vi "Test Bench v19 - TDMS.vi"() -> ()   [LabVIEW 2022 SP3]
doc: "Use this template to build a producer/consumer design pattern. Use this template when you need to execute a process, such as data analysis, when a data source, such as a triggered acquisition, produces data at an uneven rate and you need to execute the process when the data becomes available."
uses:
  <vilib>/Utility/error.llb/DialogType.ctl
  <vilib>/platform/TimedLoop/XDataNode/XDataNode.xnode
  <vilib>/Platform/TimedLoop/XDataNode/nitl_modes.ctl
  <vilib>/Platform/TimedLoop/XDataNode/XDNodeRunTimeDep.lvlib
  <vilib>/Platform/TimedLoop/XDataNode/wakeup.ctl
  <vilib>/Platform/TimedLoop/XDataNode/timing_clust.ctl
  <vilib>/measure/NI_MAPro.lvlib
  <vilib>/measure/maspectr.llb/FFT Spectrum (Mag-Phase) for 1 Chan.vi
  WhiteNoise.ctl
panel:
  in  "samples per channel":i32=41200
  in  "Folder to save file to":path=path "C:/Users/LAV-UFSC-2023/Documents/LAV-TCC/Dados-Experimentos/Dados-Bancada-LABVIEW"
  out "# pending insert":i32
  out "# pending remove":i32
  out "# elements in queue":i32
  out "Processor 2":i32=-2
  out "Iteration Duration":i64
  out "Processor":i32=-2
  out "Accelerometer":waveform(dbl)(graph)
  out "New file path":path
  in  "Log Data":bool=TRUE
  in  "view":T1={"dB On (F)"=FALSE, "unwrap phase (F)"=TRUE, "convert to degree (F)"=TRUE}
  out "FFT - Phase":cluster{"f0":dbl, "df":dbl, "phase":dbl[]}(graph)
  out "FFT - Magnitude":cluster{"f0":dbl, "df":dbl, "magnitude":dbl[]}(graph)
  out "Signal Output (V)":waveform(dbl)(graph)
  out "Iteration Duration 2":i64
  in  "Enable Output":bool=TRUE
  in  "Signal Output\nControl":enum32{"White Noise", "Harmonic"}(tab)
  in  "White Noise\nParameters":T3={"Seed"=0.0, "Standard Deviation"=2.0, "Reset"=FALSE, "Iterator"=1.0, "Lower Cut-Off"=5.0, "Upper Cut-Off"=350.0} {"Upper Cut-Off" min=5.0 max=350.0 step=10.0; "Lower Cut-Off" min=5.0 max=350.0 step=10.0; "Standard Deviation" min=0.001 max=3.0 step=0.05 format="%0.2p"}
  in  "Hamonic\nParameters":T4={"Waveform Type"=0, "Frequency (Hz)"=10.0, "Amplitude"=0.25} {"Frequency (Hz)" min=5.0 max=350.0 step=10.0 format="%0.2p"; "Waveform Type" items=["Sine Wave", "Triangle Wave", "Square Wave", "Sawtooth Wave"]; "Amplitude" min=0.001 max=0.3 step=0.05 format="%0.2p"}
  in  "stop":bool
  # "Debug Pannel"
  # "Filter"
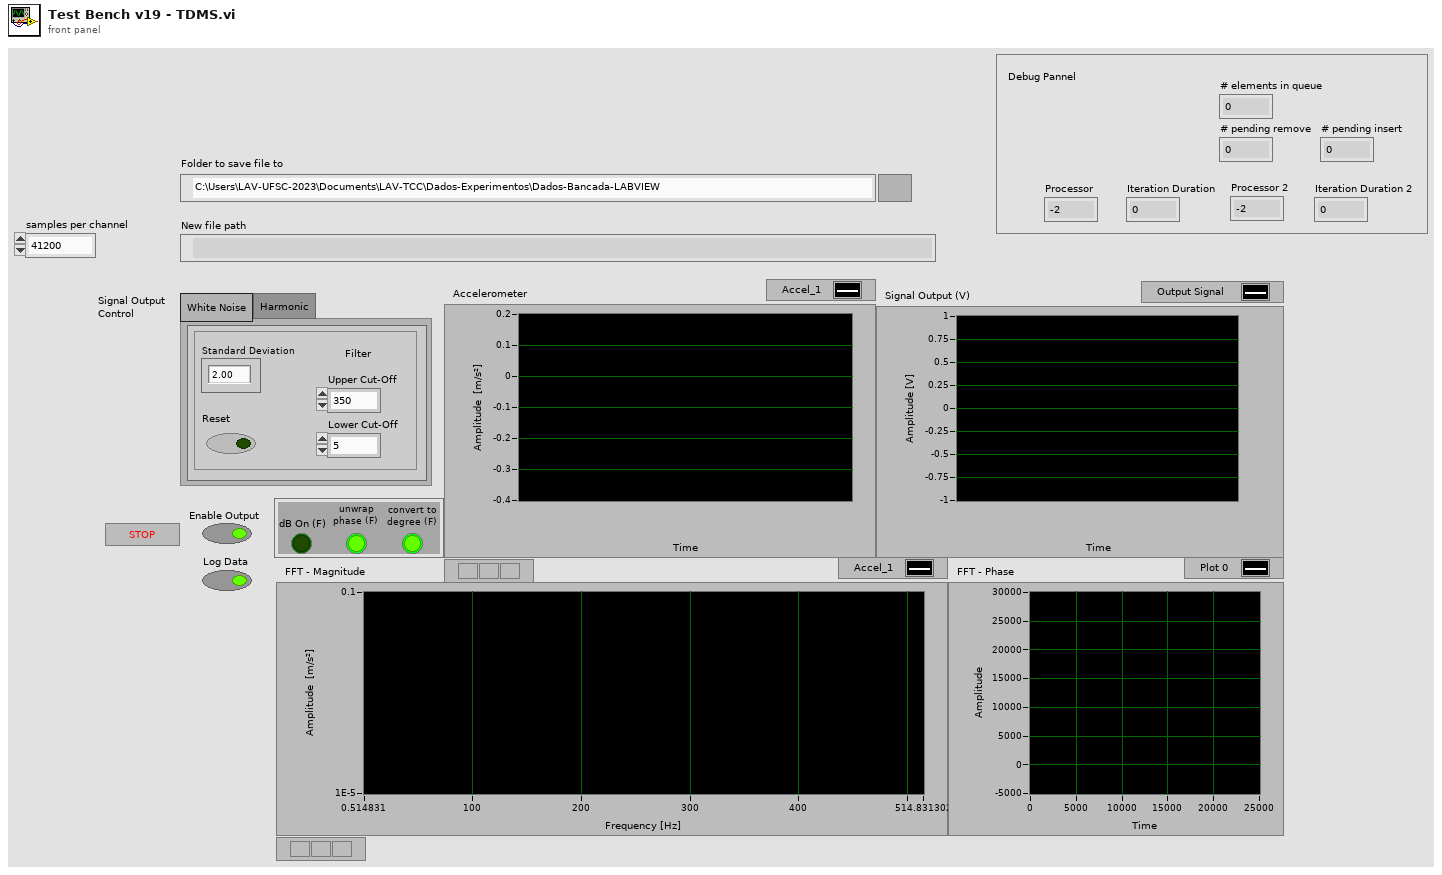
[diagram p1: front panel]
types:
  T1 = cluster{"dB On (F)":bool, "unwrap phase (F)":bool, "convert to degree (F)":bool}
  T2 = typedef "WhiteNoise.ctl" = dbl
  T3 = cluster{"Seed":T2, "Standard Deviation":dbl, "Reset":bool, "Iterator":dbl, "Lower Cut-Off":dbl, "Upper Cut-Off":dbl}
  T4 = cluster{"Waveform Type":u16, "Frequency (Hz)":dbl, "Amplitude":dbl}
  T5 = cluster{"FrameProperties":cluster{"Frame Duration":i64, "Actual Start [i]":i64}, "Accelerometer 1":waveform(dbl), "SignalOut":waveform(dbl)}
  T6 = typedef "XDNodeRunTimeDep.lvlib/timing_clust.ctl" = cluster{"Expected End [f-1]":u64, "Actual End [f-1]":u64, "Finished Late? [f-1]":bool, "Expected End [i-1]":u64, "Actual End [i-1]":u64, "Finished Late? [i-1]":bool, "Expected Start [i]":u64, "Actual Start [i]":u64, "Expected Start [f]":u64, "Actual Start [f]":u64, "Source Name":string, "Structure Name":string, "Period":i64, "Deadline":i64, "Offset":i64, "Start":i64, "Priority":i32, "Timeout":i32, "Mode":T7, "Wakeup Reason":T8, "Error":errorcluster, "Source Type":string, "Secondary Source Type":string, "Global End Time":u64, "Global Start Time":u64, "Frame Duration":u64, "Iteration Duration":u64, "Assigned CPU":i32, "I/O Scan Engine Mode":u32}
  T7 = typedef "XDNodeRunTimeDep.lvlib/nitl_modes.ctl" = enum32{"No Change", "Process missed periods, maintain original phase", "Discard missed periods, maintain original phase", "Process missed periods, ignore original phase", "Discard missed periods, ignore original phase"}
  T8 = typedef "XDNodeRunTimeDep.lvlib/wakeup.ctl" = enum32{"Normal", "Aborted", "Asynchronous wakeup", "Timing source error", "Timed loop error", "Timeout"}
  T9 = typedef "DialogType.ctl" = u16
  T10 = cluster{"Frame Duration":i64, "Actual Start [i]":i64}
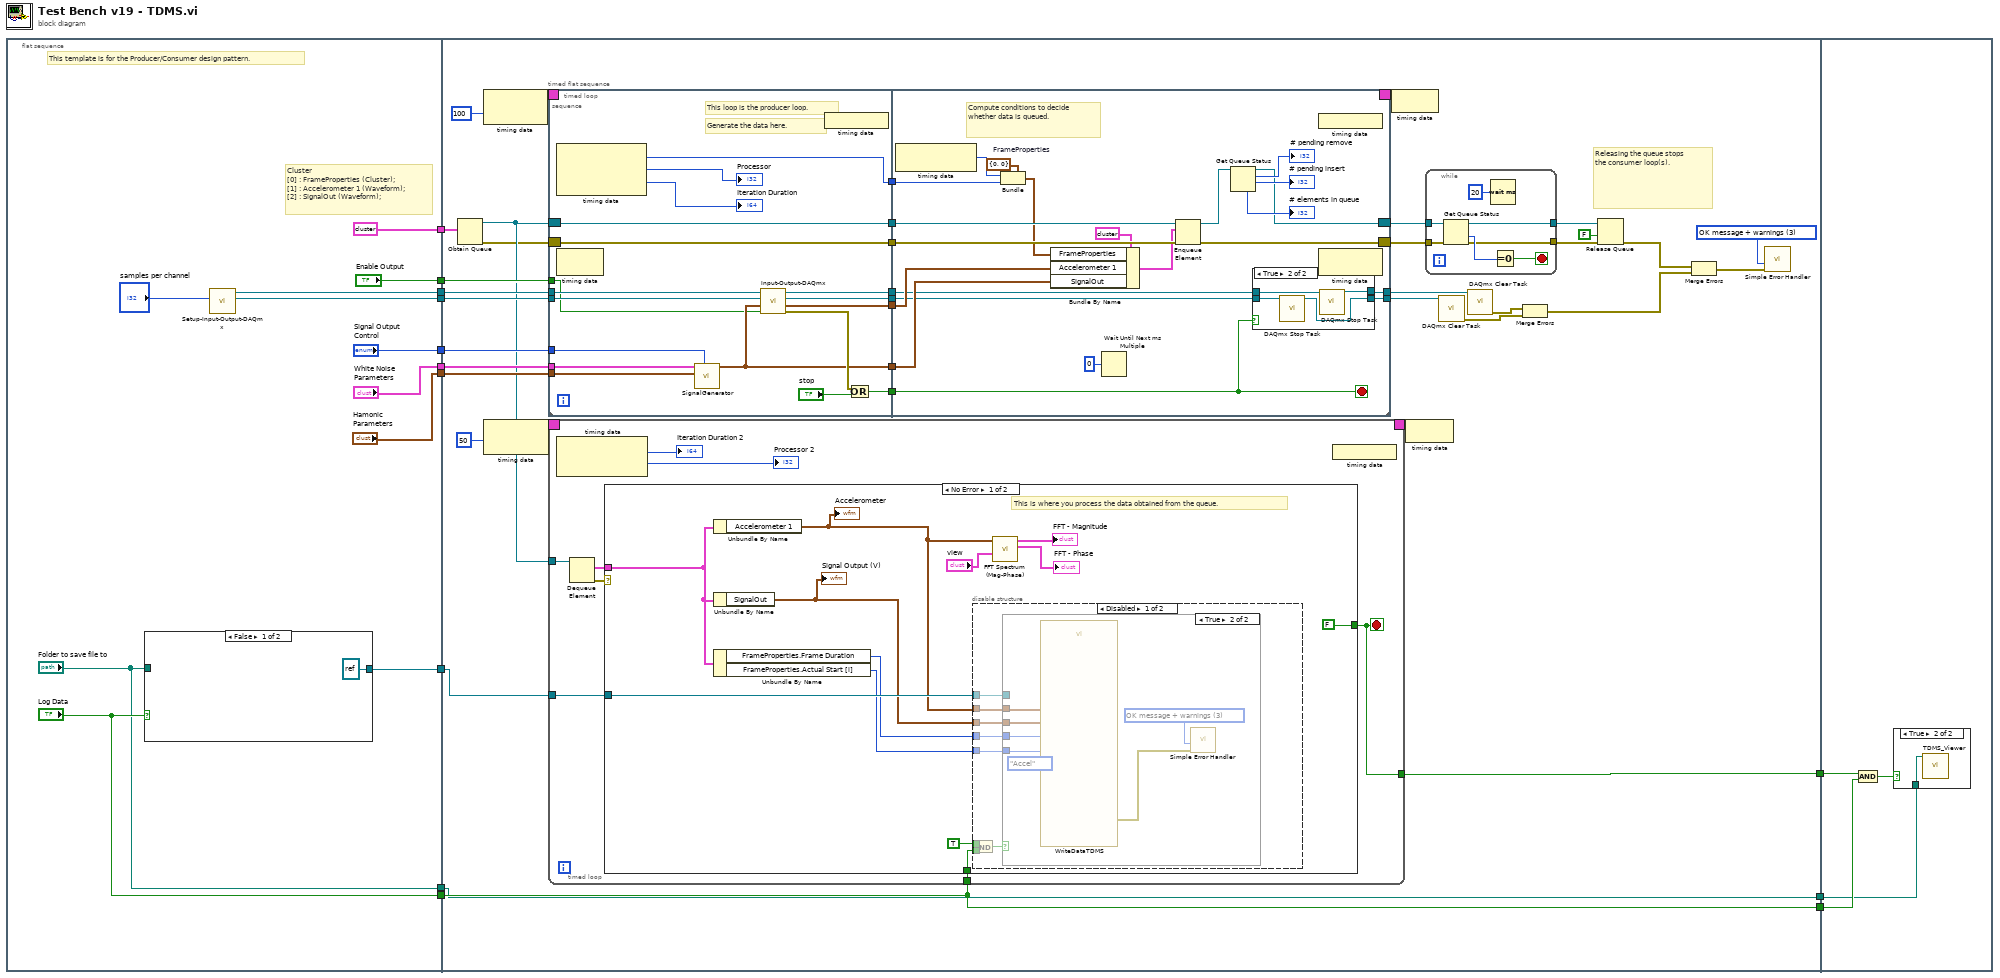
[diagram p0: block diagram]
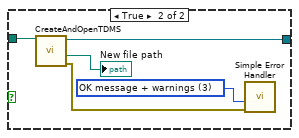
[diagram p2: hidden frame]
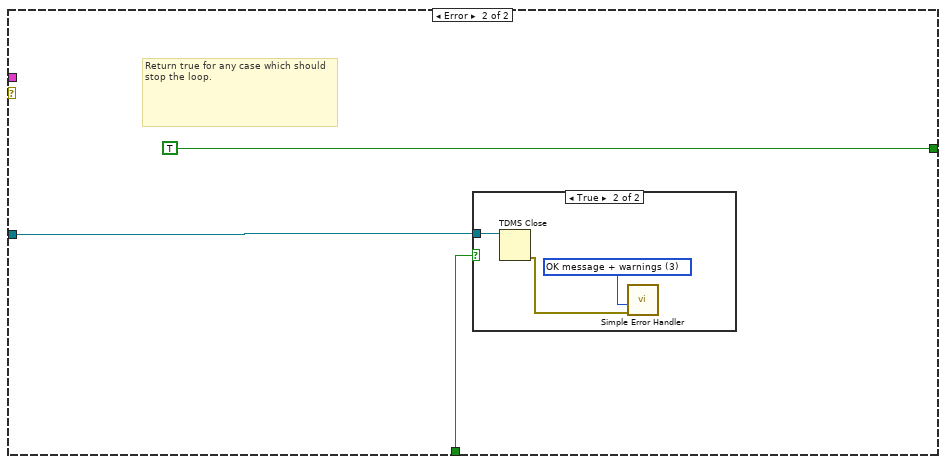
[diagram p5: hidden frame]
diagram:
  n1 = flat-sequence {
    tunnel: [w24] -> w13
    tunnel: [w23] -> w12
    tunnel: [w22] -> w11
    tunnel: ["Log Data"] -> w10
    tunnel: ["Folder to save file to"] -> w6
    tunnel: ["Signal Output\nControl"] -> w5
    tunnel: ["Enable Output"] -> w4
    tunnel: ["White Noise\nParameters"] -> w3
    tunnel: ["Hamonic\nParameters"] -> w2
    tunnel: [T5 {"FrameProperties"={"Frame Duration"=0, "Actual Start [i]"=0}, "Accelerometer 1"={"t0"=timestamp(0 s since 1904-01-01), "dt"=1.0, "Y"=[]}, "SignalOut"={"t0"=timestamp(0 s since 1904-01-01), "dt"=1.0, "Y"=[]}} ("input cluster")] -> w1
    tunnel: w13 -> [w57]
    tunnel: w12 -> [w56]
    tunnel: w11 -> [w52]
    tunnel: w10 -> [w50]
    tunnel: [w50] -> w9
    tunnel: [w49] -> w8
    tunnel: [w48] -> w7
    tunnel: w6 -> [w48]
    tunnel: w5 -> [w37]
    tunnel: w4 -> [w36]
    tunnel: w3 -> [w35]
    tunnel: w2 -> [w34]
    tunnel: w1 -> [w33]
    tunnel: w7 -> [w212]
    tunnel: w8 -> [w211]
    tunnel: w9 -> [w213]
    frame #0 {
      # "Cluster\n[0] : FrameProperties (Cluster);\n[1] : Accelerometer 1 (Waveform);\n[2] : SignalOut (Waveform);"
      # "This template is for the Producer/Consumer design pattern."
      n2 = case shown="False" "Log Data" {
        tunnel: [refnum<k34> refnum ("tdms file out") w27] -> w22
        tunnel: "Folder to save file to" -> [_ w26]
        frame False {
        }
        frame True {
          w29 = T9 3 items=["no dialog", "OK message", "continue or stop message", "OK message + warnings", "continue/stop + warnings"] ("type of dialog (OK msg:1)")
          n3 = call "CreateAndOpenTDMS.vi"("Folder to save file to"=w26) -> ("error out"=w30:errorcluster, "New file path"=→"New file path":path, "tdms file out"=w27:refnum<k34>)  [unwired: 8 in]
          n4 = call <vilib>:"Simple Error Handler.vi"("type of dialog (OK msg:1)"=w29, "error in (no error)"=w30) -> ()  [unwired: 3 in, 5 out]
        }
      }
      n5 = call "Setup-Input-Output-DAQmx.vi"("samples per channel"="samples per channel") -> ("Output task"=w23:refnum<k21>, "Input Task"=w24:refnum<k21>)  [unwired: 8 in, 1 out]
    }
    frame #1 {
      w39 = T9 3 items=["no dialog", "OK message", "continue or stop message", "OK message + warnings", "continue/stop + warnings"] ("type of dialog (OK msg:1)")
      # "Releasing the queue stops the consumer loop(s)."
      n6 = Obtain Queue(element data type=w33) -> (queue out=w32:refnum<queue>, error out=w31:errorcluster)  [unwired: 4 in, 1 out]
      n7 = node-c288(100 ("Priority")) -> (w62:T6)
      n8 = node-c288(50 ("Priority")) -> (w60:T6)
      n9 = timed-loop {
        shift-right: [w123] -> w47
        shift-left: w31 -> [w128]
        shift-right: [w126] -> w51
        shift-left: w32 -> [w127]
        tunnel: [w124] -> w54
        tunnel: [w125] -> w55
        tunnel: w57 -> [w130]
        tunnel: w56 -> [w129]
        timing: w62 -> [_]
        timing-out: [_] -> w61
        tunnel: w37 -> [w122]
        tunnel: w36 -> [w121]
        tunnel: w35 -> [w120]
        tunnel: w34 -> [w119]
        stop <- w179 stop-if-true
        n10 = timed-sequence {
          timing: _ -> [_]
          timing-out: _ -> [_]
          tunnel: w130 -> [w150]
          tunnel: w129 -> [w149]
          tunnel: w128 -> [w148]
          tunnel: w127 -> [w147]
          tunnel: [w146] -> w126
          tunnel: [w137] -> w125
          tunnel: [w136] -> w124
          tunnel: [w135] -> w123
          tunnel: w122 -> [w134]
          tunnel: w121 -> [w133]
          tunnel: w120 -> [w132]
          tunnel: w119 -> [w131]
          n11 = timed-flat-sequence {
            tunnel: w150 -> [w166]
            tunnel: w149 -> [w165]
            tunnel: w148 -> [w161]
            tunnel: w147 -> [w160]
            tunnel: [w168] -> w145
            tunnel: [w167] -> w144
            tunnel: [w161] -> w143
            tunnel: [w160] -> w142
            tunnel: [w164] -> w141
            tunnel: [w159] -> w140
            tunnel: [w155] -> w139
            tunnel: [w158] -> w138
            tunnel: w134 -> [w154]
            tunnel: w133 -> [w153]
            tunnel: w132 -> [w152]
            tunnel: w131 -> [w151]
            tunnel: [w180] -> w146
            tunnel: w145 -> [w177]
            tunnel: w144 -> [w178]
            tunnel: w143 -> [w195]
            tunnel: w142 -> [w193]
            tunnel: w141 -> [w179]
            tunnel: w140 -> [w191]
            tunnel: w139 -> [w190]
            tunnel: w138 -> [w189]
            tunnel: [w176] -> w137
            tunnel: [w175] -> w136
            tunnel: [w194] -> w135
            frame #0 {
              # "Generate the data here."
              # "This loop is the producer loop."
              n12 = node-c288() -> (w159:i64, →"Processor":i32, →"Iteration Duration":i64)  [unwired: 1 in]
              n13 = call "SignalGenerator.vi"("Signal Output\nControl"=w154, "Hamonic\nParameters"=w151, "White Noise\nParameters"=w152) -> ("Signal Out"=w155:waveform(dbl))  [unwired: 8 in]
              n14 = call "Input-Output-DAQmx.vi"("Enable Output"=w153, "data"=w155, "task/channels in"=w165, "Input Task In"=w166) -> ("error out"=w162:errorcluster, "Input Data Sink"=w158:waveform(dbl), "task out"=w168:refnum<k21>, "Input task Out"=w167:refnum<k21>)  [unwired: 4 in]
              n15 = node-c288() -> ()  [unwired: 1 out]
              n16 = Or(x=w162, y="stop") -> (x .or. y?=w164:bool)
            }
            frame #1 {
              w186 = T10 {"Frame Duration"=0, "Actual Start [i]"=0}  # FrameProperties
              # "Compute conditions to decide whether data is queued."
              n17 = node-c288() -> (w192:i64)  [unwired: 1 in]
              n18 = Bundle(cluster=w186, "Frame Duration"=w192, "Actual Start [i]"=w191) -> (w187:T10)
              n19 = Bundle By Name(cluster=T5 {"FrameProperties"={"Frame Duration"=0, "Actual Start [i]"=0}, "Accelerometer 1"={"t0"=timestamp(0 s since 1904-01-01), "dt"=1.0, "Y"=[]}, "SignalOut"={"t0"=timestamp(0 s since 1904-01-01), "dt"=1.0, "Y"=[]}} ("input cluster"), "FrameProperties"=w187, "Accelerometer 1"=w189, "SignalOut"=w190) -> (w188:T5)
              n20 = Wait Until Next ms Multiple(millisecond multiple=u32 0) -> ()  [unwired: 1 out]
              n21 = Enqueue Element(queue=w193, element=w188, error in (no error)=w195) -> (queue out=w181:refnum<queue>, error out=w194:errorcluster)  [unwired: 1 in, 1 out]
              n22 = Get Queue Status(queue=w181) -> (queue out=w180:refnum<queue>, # pending remove=→"# pending remove":i32, # pending insert=→"# pending insert":i32, # elements in queue=→"# elements in queue":i32)  [unwired: 2 in, 4 out]
              n23 = case shown="True" w179 {
                tunnel: [w196 w201] -> w176
                tunnel: w178 -> [w196 w200]
                tunnel: w177 -> [w197 w199]
                tunnel: [w197 w198] -> w175
                frame False {
                }
                frame True {
                  n24 = call <vilib>:"DAQmx Stop Task.vi"("task/channels in"=w199) -> ("task out"=w198:refnum<k21>)  [unwired: 13 in, 1 out]
                  n25 = call <vilib>:"DAQmx Stop Task.vi"("task/channels in"=w200) -> ("task out"=w201:refnum<k21>)  [unwired: 13 in, 1 out]
                }
              }
              n26 = node-c288() -> ()  [unwired: 1 out]
            }
          }
        }
        n27 = node-c288() -> ()  [unwired: 1 in, 1 out]
        n28 = node-c288() -> ()  [unwired: 1 in, 1 out]
      }
      n29 = timed-loop {
        tunnel: w32 -> [w77]
        timing: w60 -> [_]
        timing-out: [_] -> w59
        tunnel: w50 -> [w72]
        tunnel: [w70] -> w49
        tunnel: w52 -> [w73]
        stop <- w70 stop-if-true
        n30 = node-c288() -> (→"Iteration Duration 2":i64, →"Processor 2":i32)  [unwired: 1 in]
        n31 = Dequeue Element(queue=w77) -> (element=w75:T5, error out=w76:errorcluster)  [unwired: 2 in, 2 out]
        n32 = case shown="No Error" w76 {
          tunnel: w75 -> [w89 _]
          tunnel: [FALSE TRUE] -> w70
          tunnel: w73 -> [w90 w109]
          tunnel: w72 -> [w83 w110]
          frame No Error {
            # "This is where you process the data obtained from the queue."
            n33 = Unbundle By Name(w89) -> ("Accelerometer 1"=w88:waveform(dbl))
            "Accelerometer" <- w88
            n34 = Unbundle By Name(w89) -> ("SignalOut"=w87:waveform(dbl))
            "Signal Output (V)" <- w87
            n35 = Unbundle By Name(w89) -> ("FrameProperties.Frame Duration"=w86:i64, "FrameProperties.Actual Start [i]"=w85:i64)
            n36 = disable-structure shown="Disabled" {
              disable-tunnel: w90 -> [w101 _]
              disable-tunnel: w88 -> [w100 _]
              disable-tunnel: w87 -> [w99 _]
              disable-tunnel: w86 -> [w98 _]
              disable-tunnel: w85 -> [w97 _]
              disable-tunnel: w83 -> [w95 _]
              disable-tunnel: TRUE ("x") -> [w94 _]
              frame Disabled {
                n37 = And(x=w94, y=w95) -> (x .and. y?=w96:bool)
                n38 = case shown="True" w96 {
                  tunnel: w101 -> [_ _]
                  tunnel: w100 -> [_ w106]
                  tunnel: w99 -> [_ w105]
                  tunnel: w98 -> [_ w104]
                  tunnel: w97 -> [_ w103]
                  frame False {
                  }
                  frame True {
                    w108 = T9 3 items=["no dialog", "OK message", "continue or stop message", "OK message + warnings", "continue/stop + warnings"] ("type of dialog (OK msg:1)")
                    n39 = call "WriteDataTDMS.vi"("SignalOut"=w105, "Accel."=w106, "Identifier"=enum16{"Accel", "SignalOut", "ButtonPress"}."Accel", "TimeInterval"=w104, "ActualStart[f]"=w103) -> ("error out"=w107:errorcluster)  [unwired: 21 in, 1 out]
                    n40 = call <vilib>:"Simple Error Handler.vi"("type of dialog (OK msg:1)"=w108, "error in (no error)"=w107) -> ()  [unwired: 3 in, 5 out]
                  }
                }
              }
              frame Enabled {
              }
            }
            n41 = call-poly <vilib>:"FFT Spectrum (Mag-Phase).vi"("view"="view", "time signal"=w88) -> ("phase"=→"FFT - Phase":cluster{"f0":dbl, "df":dbl, "phase":dbl[]}, "magnitude"=→"FFT - Magnitude":cluster{"f0":dbl, "df":dbl, "magnitude":dbl[]})  [unwired: 5 in, 3 out]
          }
          frame Error {
            # "Return true for any case which should stop the loop."
            n42 = case shown="True" w110 {
              tunnel: w109 -> [_ w113]
              frame False {
              }
              frame True {
                w114 = T9 3 items=["no dialog", "OK message", "continue or stop message", "OK message + warnings", "continue/stop + warnings"] ("type of dialog (OK msg:1)")
                n43 = TDMS Close(11:w113) -> (0:w112:errorcluster)  [unwired: 1 in, 1 out]
                n44 = call <vilib>:"Simple Error Handler.vi"("type of dialog (OK msg:1)"=w114, "error in (no error)"=w112) -> ()  [unwired: 3 in, 5 out]
              }
            }
          }
        }
        n45 = node-c288() -> ()  [unwired: 1 out]
      }
      n46 = node-c288(w61) -> ()
      n47 = node-c288(w59) -> ()
      n48 = while {
        tunnel: w47 -> [w69]
        tunnel: w51 -> [w68]
        tunnel: [w65] -> w46
        tunnel: [w64] -> w45
        stop <- w66 stop-if-true
        n49 = Get Queue Status(queue=w68, error in (no error)=w69) -> (queue out=w64:refnum<queue>, # pending insert=w67:i32, error out=w65:errorcluster)  [unwired: 1 in, 5 out]
        n50 = Wait (ms)(milliseconds to wait=u32 20) -> ()  [unwired: 1 out]
        n51 = Equal To 0?(x=w67) -> (x = 0?=w66:bool)
      }
      n52 = call <vilib>:"DAQmx Clear Task.vi"("task in"=w54) -> ("error out"=w43:errorcluster)  [unwired: 14 in]
      n53 = call <vilib>:"DAQmx Clear Task.vi"("task in"=w55) -> ("error out"=w44:errorcluster)  [unwired: 14 in]
      n54 = Merge Errors(w44, w43) -> (w40:errorcluster)
      n55 = Release Queue(queue=w45, force destroy? (F)=FALSE, error in (no error)=w46) -> (error out=w41:errorcluster)  [unwired: 2 out]
      n56 = Merge Errors(w41, w40) -> (w42:errorcluster)
      n57 = call <vilib>:"Simple Error Handler.vi"("type of dialog (OK msg:1)"=w39, "error in (no error)"=w42) -> ()  [unwired: 3 in, 5 out]
    }
    frame #2 {
      n58 = And(x=w211, y=w213) -> (x .and. y?=w214:bool)
      n59 = case shown="True" w214 {
        tunnel: w212 -> [_ w215]
        frame False {
        }
        frame True {
          n60 = call "TDMS_Viewer.vi"("Data Directory"=w215) -> ()  [unwired: 11 in]
        }
      }
    }
  }
